vi "Lado e Cor.vi"(9 "Field Size 2":T4, 10 "Game Status":T6 {"Time" format="%<%.3X %x>T"; "Blue Timeout Remaining" format="%<%M:%S>t"; "Yellow Timeout Remaining" format="%<%M:%S>t"; "Time Left" format="%<%M:%S>t"}, 11 "Input Detection Frame":T7) -> (3 "Output IA Input":T1)   [LabVIEW 2016]
uses:
  SSL Detection Robot.ctl
  SSL Detection Ball.ctl
  SSL Referee Game Status.ctl
  Field Size.ctl
  IA Input.ctl
  IA Judge.ctl
panel:
  in  "Lado":enum16{"Esquerdo", "Direito"}(ring) caption="Enum"
  in  "Time":enum16{"Azul", "Amarelo"}(ring) caption="Enum"
  # "Score"
  # "Red Cards"
  # "Yellow Cards"
  # "Timeouts Left"
  # "Timeout Remaining"
  # "Goalie ID"
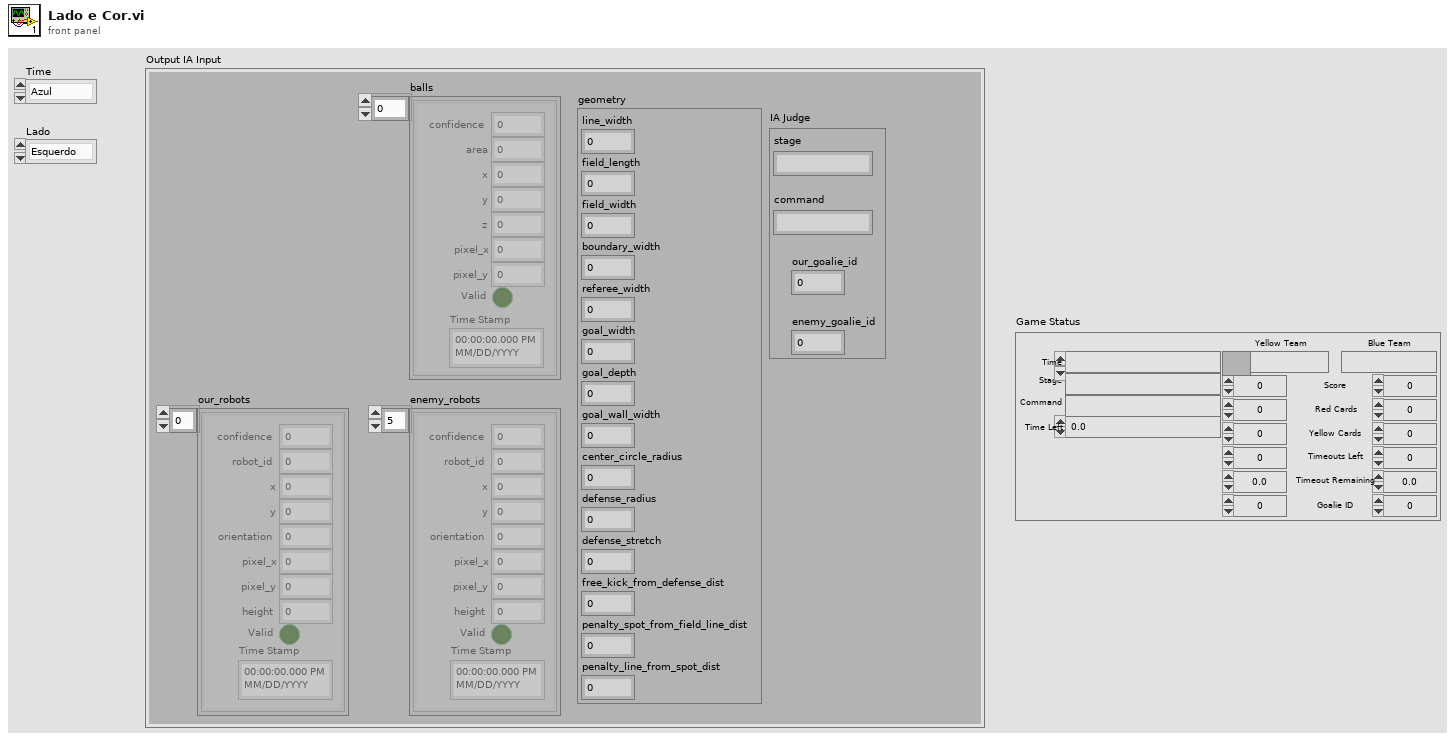
[diagram p1: front panel]
types:
  T1 = typedef "IA Input.ctl" = cluster{"our_robots":T2[], "enemy_robots":T2[], "balls":T3[], "geometry":T4, "IA Judge":T5}
  T2 = typedef "SSL Detection Robot.ctl" = cluster{"x":dbl, "robot_id":u32, "confidence":sgl, "y":sgl, "orientation":sgl, "pixel_x":sgl, "pixel_y":sgl, "height":sgl, "Valid":bool, "Time Stamp":timestamp}
  T3 = typedef "SSL Detection Ball.ctl" = cluster{"x":sgl, "area":u32, "confidence":sgl, "y":sgl, "z":sgl, "pixel_x":sgl, "pixel_y":sgl, "Valid":bool, "Time Stamp":timestamp}
  T4 = typedef "Field Size.ctl" = cluster{"line_width":u32, "field_length":u32, "field_width":u32, "boundary_width":u32, "referee_width":u32, "goal_width":u32, "goal_depth":u32, "goal_wall_width":u32, "center_circle_radius":u32, "defense_radius":u32, "defense_stretch":u32, "free_kick_from_defense_dist":u32, "penalty_spot_from_field_line_dist":u32, "penalty_line_from_spot_dist":u32}
  T5 = typedef "IA Judge.ctl" = cluster{"stage":string, "command":string, "our_goalie_id":dbl, "enemy_goalie_id":dbl}
  T6 = typedef "SSL Referee Game Status.ctl" = cluster{"Stage":string, "Command":string, "Time Left":dbl, "Yellow Team":string, "Blue Team":string, "Yellow Score":u32, "Blue Score":u32, "Yellow Red Cards":u32, "Blue Red Cards":u32, "Yellow Yellow Cards":u32, "Blue Yellow Cards":u32, "Yellow Timeouts Left":u32, "Blue Timeouts Left":u32, "Yellow Timeout Remaining":dbl, "Blue Timeout Remaining":dbl, "Yellow Goalie Id":u32, "Blue Goalie Id":u32, "Time":timestamp}
  T7 = cluster{"frame_number":u32, "t_capture":dbl, "t_sent":dbl, "camera_id":u32, "robots_yellow":T2[], "robots_blue":T2[], "balls":T3[], "Valid":bool, "Time Stamp":timestamp}
  T8 = typedef "SSL Detection Frame.ctl" = cluster{"frame_number":u32, "t_capture":dbl, "t_sent":dbl, "camera_id":u32, "robots_yellow":T2[], "robots_blue":T2[], "balls":T3[], "Valid":bool, "Time Stamp":timestamp}
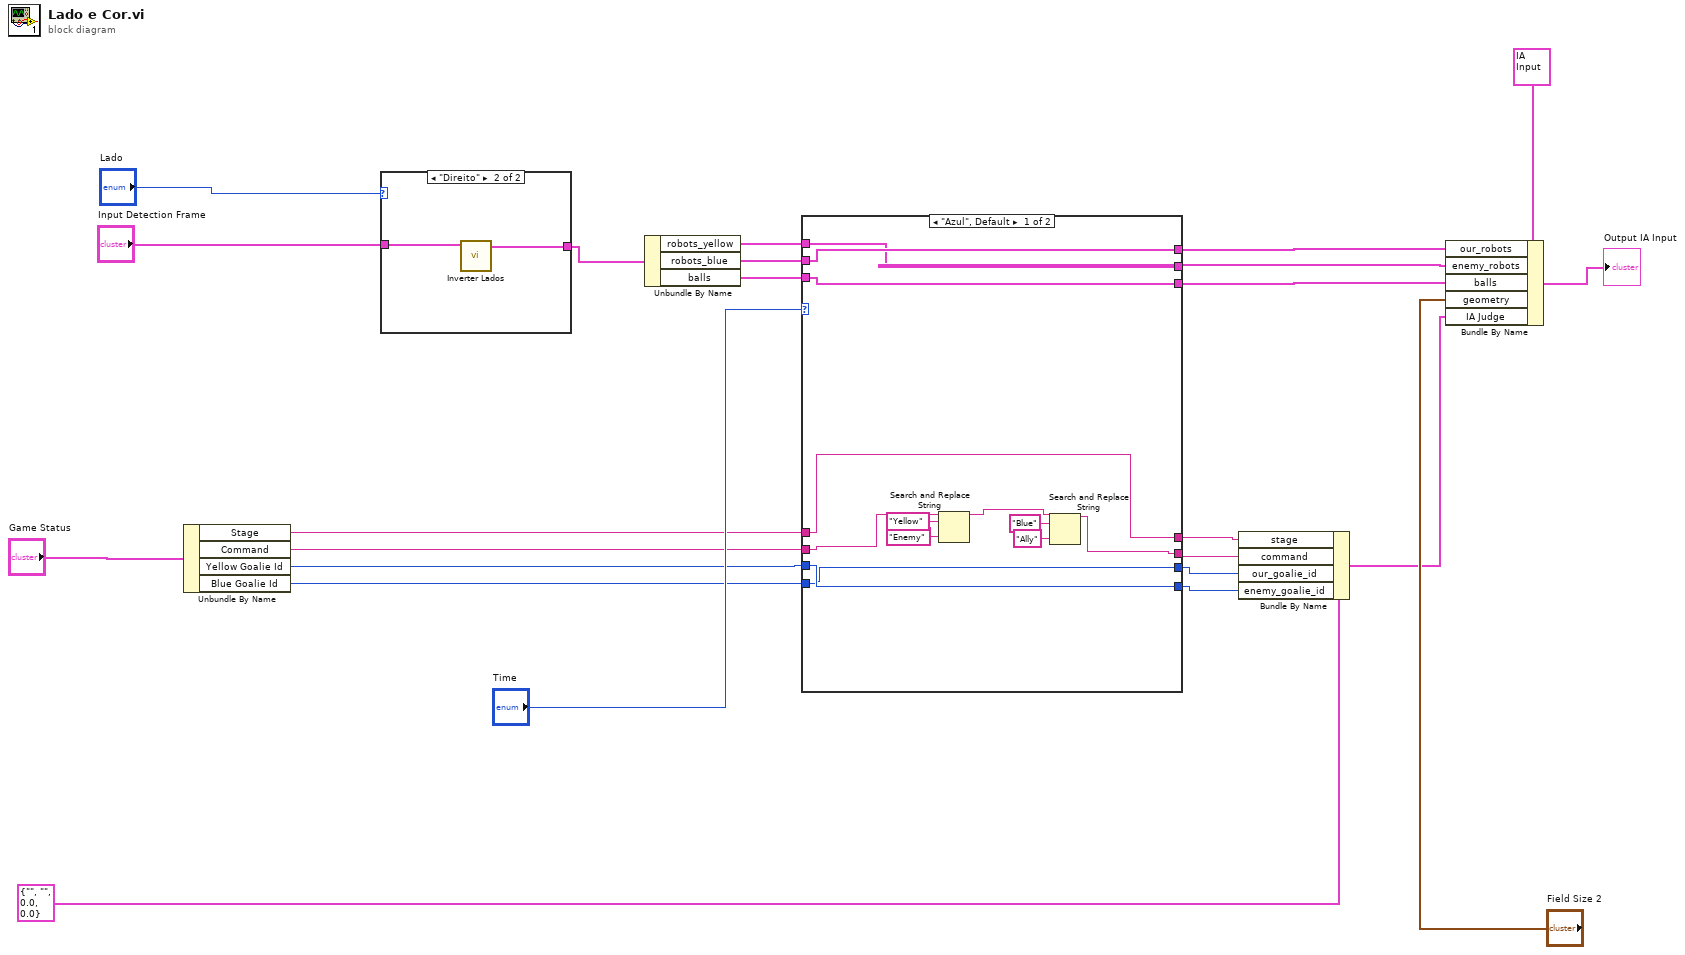
[diagram p0: block diagram]
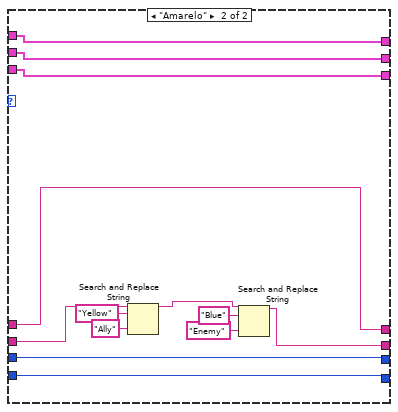
[diagram p2: hidden frame]
diagram:
  n1 = Unbundle By Name("Game Status") -> ("Stage"=w6:string, "Command"=w5:string, "Yellow Goalie Id"=w10:u32, "Blue Goalie Id"=w9:u32)
  n2 = case shown="\"Direito\"" "Lado" {
    tunnel: "Input Detection Frame" -> [w25 w27]
    tunnel: [w25 w26] -> w20
    frame "Esquerdo", Default {
    }
    frame "Direito" {
      n3 = call "Inverter Lados.vi"("Detection Frame"=w27) -> ("output cluster"=w26:T8)  [unwired: 10 in]
    }
  }
  n4 = Unbundle By Name(w20) -> ("robots_yellow"=w19:T2[], "robots_blue"=w18:T2[], "balls"=w17:T3[])
  n5 = case shown="\"Azul\", Default" "Time" {
    tunnel: w19 -> [w39 w51]
    tunnel: w18 -> [w40 w52]
    tunnel: w17 -> [w38 w53]
    tunnel: [w40 w51] -> w16
    tunnel: [w39 w52] -> w15
    tunnel: [w38 w53] -> w14
    tunnel: w10 -> [w37 w50]
    tunnel: w9 -> [w36 w49]
    tunnel: [w37 w49] -> w3
    tunnel: [w36 w50] -> w4
    tunnel: w6 -> [w28 w48]
    tunnel: w5 -> [w30 w47]
    tunnel: [w28 w48] -> w2
    tunnel: [w29 w41] -> w1
    frame "Azul", Default {
      n6 = Search and Replace String(input string=w30, search string="Yellow", replace string="Enemy" ("replace string (\"\")")) -> (result string=w35:string)  [unwired: 5 in, 3 out]
      n7 = Search and Replace String(input string=w35, search string="Blue", replace string="Ally" ("replace string (\"\")")) -> (result string=w29:string)  [unwired: 5 in, 3 out]
    }
    frame "Amarelo" {
      n8 = Search and Replace String(input string=w47, search string="Yellow", replace string="Ally" ("replace string (\"\")")) -> (result string=w42:string)  [unwired: 5 in, 3 out]
      n9 = Search and Replace String(input string=w42, search string="Blue", replace string="Enemy" ("replace string (\"\")")) -> (result string=w41:string)  [unwired: 5 in, 3 out]
    }
  }
  n10 = Bundle By Name(cluster=T5 {"stage"="", "command"="", "our_goalie_id"=0.0, "enemy_goalie_id"=0.0} ("IA Judge"), "stage"=w2, "command"=w1, "our_goalie_id"=w4, "enemy_goalie_id"=w3) -> (w8:T5)
  n11 = Bundle By Name(cluster=T1 {"our_robots"=[], "enemy_robots"=[], "balls"=[], "geometry"={"line_width"=0, "field_length"=0, "field_width"=0, "boundary_width"=0, "referee_width"=0, "goal_width"=0, "goal_depth"=0, "goal_wall_width"=0, "center_circle_radius"=0, "defense_radius"=0, "defense_stretch"=0, "free_kick_from_defense_dist"=0, "penalty_spot_from_field_line_dist"=0, "penalty_line_from_spot_dist"=0}, "IA Judge"={"stage"="", "command"="", "our_goalie_id"=0.0, "enemy_goalie_id"=0.0}} ("Detection Frame"), "our_robots"=w16, "enemy_robots"=w15, "balls"=w14, "geometry"="Field Size 2", "IA Judge"=w8) -> (→"Output IA Input":T1)
